vi "Calculate&Save.vi"(9 "机械手":dbl[](array[numeric]), 10 "像素":dbl[](array[numeric])) -> ()   [LabVIEW 2016]
uses:
  <vilib>/Utility/config.llb/Write Key (String).vi
  <vilib>/Utility/config.llb/Write Key (Double).vi
  <vilib>/Utility/config.llb/NI_LVConfig.lvlib
panel:
  out "error out":errorcluster caption="错误输出"
  in  "error in (no error)":errorcluster caption="错误输入（无错误）"
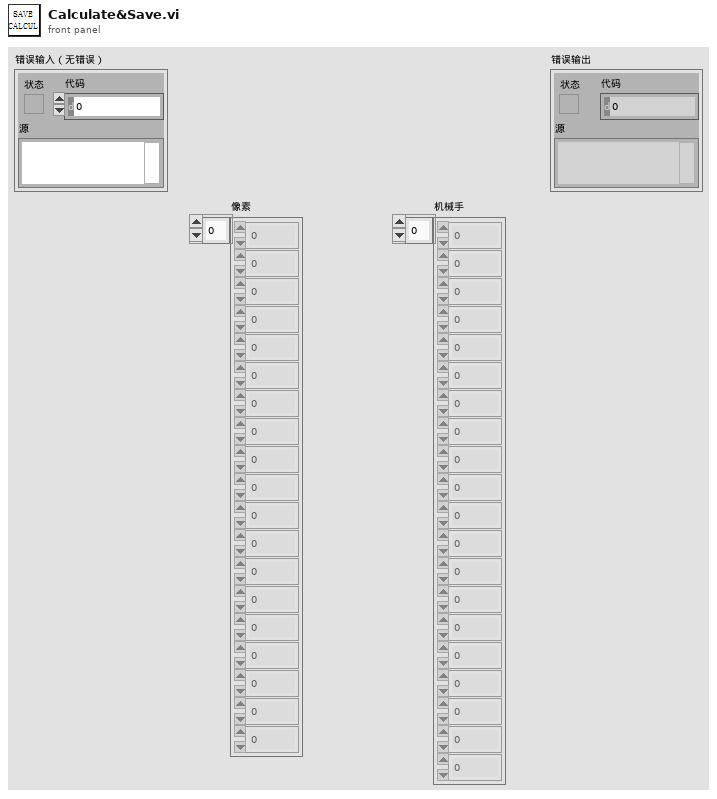
[diagram p1: front panel]
types:
  T1 = typedef "NI_LVConfig.lvlib/Config Data RefNum.ctl" = refnum<k1>
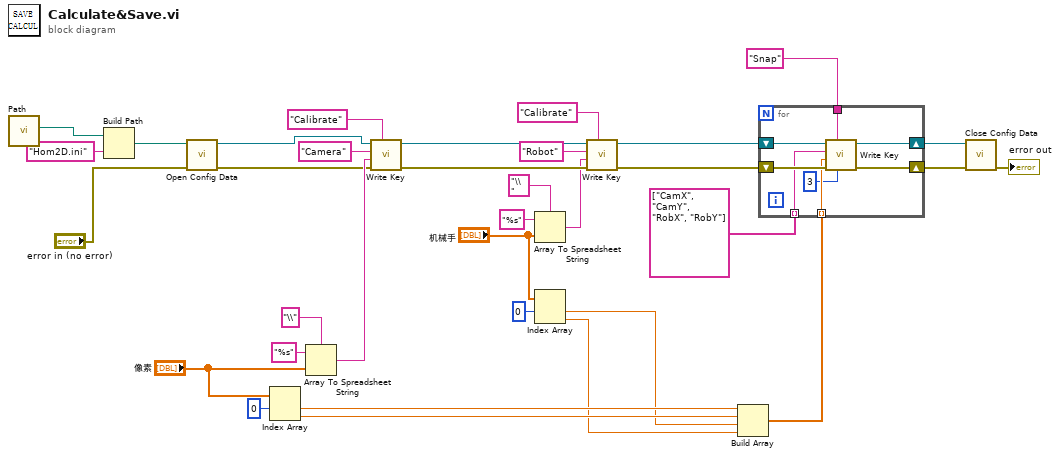
[diagram p0: block diagram]
diagram:
  n1 = call "Path.vi"() -> ("Total"=w34:path)  [unwired: 11 in]
  n2 = Build Path(base path=w34, name or relative path="Hom2D.ini" ("名称或相对路径")) -> (appended path=w32:path)
  n3 = call <vilib>:"Open Config Data.vi"("error in (no error)"="error in (no error)", "configuration file path"=w32) -> ("error out"=w10:errorcluster, "refnum"=w11:T1)  [unwired: 7 in, 1 out]
  n4 = Index Array(array="像素", index #1=0 ("索引")) -> (element #1=w5:dbl, element #2=w4:dbl)  [unwired: 1 in]
  n5 = Array To Spreadsheet String(delimiter (Tab)="\\" ("分隔符(Tab)"), array="像素", 3:"%s" ("格式字符串")) -> (spreadsheet string=w25:string)
  n6 = call-poly <vilib>:"Write Key.vi"("section"="Calibrate", "error in (no error)"=w10, "value"=w25, "key"="Camera" ("section"), "refnum"=w11) -> ("error out"=w30:errorcluster, "refnum out"=w31:T1)  [unwired: 4 in, 1 out]
  n7 = Array To Spreadsheet String(delimiter (Tab)="\\ " ("分隔符(Tab)"), array="机械手", 3:"%s" ("格式字符串")) -> (spreadsheet string=w22:string)
  n8 = Index Array(array="机械手", index #1=0 ("索引")) -> (element #1=w3:dbl, element #2=w2:dbl)  [unwired: 1 in]
  n9 = call-poly <vilib>:"Write Key.vi"("section"="Calibrate", "error in (no error)"=w30, "value"=w22, "key"="Robot" ("section"), "refnum"=w31) -> ("error out"=w9:errorcluster, "refnum out"=w8:T1)  [unwired: 4 in, 1 out]
  n10 = Build Array(w5, w4, w3, w2) -> (w1:dbl[])
  n11 = for {
    tunnel: "Snap" ("section") -> [w40]
    shift-right: [w41] -> w7
    shift-left: w8 -> [w42]
    shift-right: [w38] -> w6
    shift-left: w9 -> [w39]
    tunnel: string[] ["CamX", "CamY", "RobX", "RobY"] -> [w37] mode=indexing
    tunnel: w1 -> [w36] mode=indexing
    n12 = call-poly <vilib>:"Write Key.vi"("precision (6)"=i16 3, "section"=w40, "error in (no error)"=w39, "value"=w36, "key"=w37, "refnum"=w42) -> ("error out"=w38:errorcluster, "refnum out"=w41:T1)  [unwired: 3 in, 1 out]
  }
  n13 = call <vilib>:"Close Config Data.vi"("error in (no error)"=w6, "refnum"=w7) -> ("error out"=→"error out":errorcluster)  [unwired: 8 in, 1 out]
